vi "Update Position Simple.vi"(2 "error in (no error)":errorcluster, 3 "Time Since Last Update":dbl, 4 "Car.lvclass":refnum<class "Car.lvclass">) -> (0 "error out":errorcluster, 1 "Car.lvclass 2":refnum<class "Car.lvclass">)   [LabVIEW 2015, in "Car.lvclass"]
uses:
  Car.lvclass
  Car.lvclass/Car.ctl
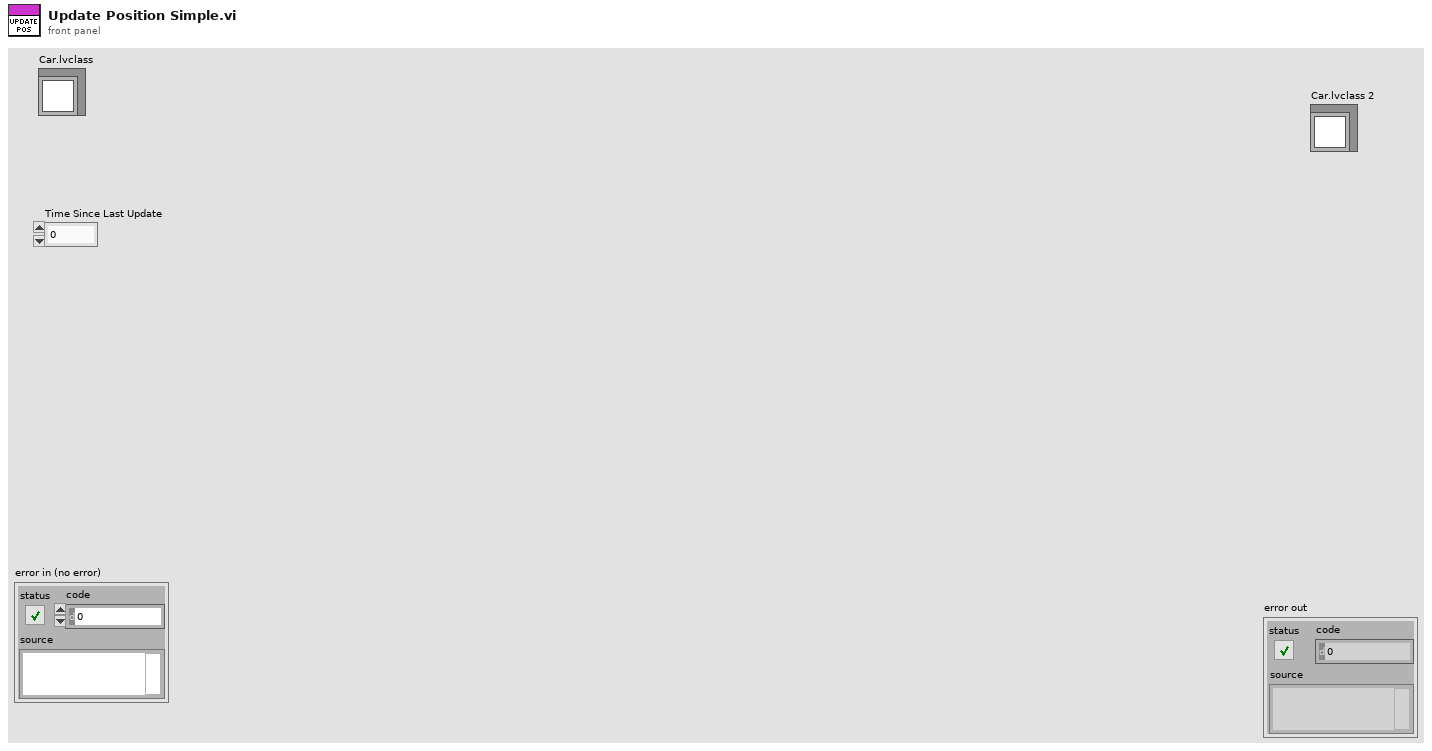
[diagram p1: front panel]
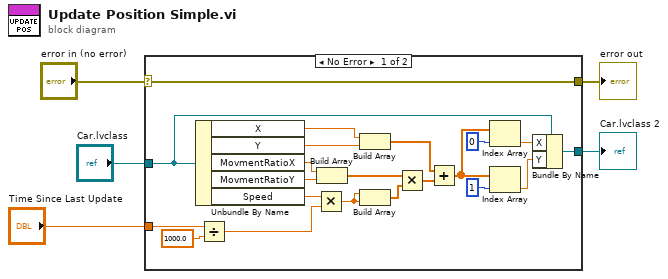
[diagram p0: block diagram]
diagram:
  n1 = case shown="No Error" "error in (no error)" {
    selector: "error in (no error)" -> [w26 w28]
    tunnel: [w26 w28] -> w4
    tunnel: [w12 w27] -> w3
    tunnel: "Car.lvclass" -> [w18 w27]
    tunnel: "Time Since Last Update" -> [w11 _]
    frame No Error {
      n2 = Unbundle By Name(w18) -> ("X"=w7:dbl, "Y"=w6:dbl, "MovmentRatioX"=w24:dbl, "MovmentRatioY"=w23:dbl, "Speed"=w8:dbl)
      n3 = Divide(x=w11, y=1000.0) -> (x/y=w9:dbl)
      n4 = Multiply(x=w8, y=w9) -> (x*y=w25:dbl)
      n5 = Build Array(w24, w23) -> (w22:dbl[])
      n6 = Build Array(w7, w6) -> (w20:dbl[])
      n7 = Build Array(w25, w25) -> (w21:dbl[])
      n8 = Multiply(x=w22, y=w21) -> (x*y=w19:dbl[])
      n9 = Add(x=w20, y=w19) -> (x+y=w13:dbl[])
      n10 = Index Array(array=w13, index=0) -> (element=w14:dbl)
      n11 = Index Array(array=w13, index=1) -> (element=w15:dbl)
      n12 = Bundle By Name(cluster=w18, "X"=w14, "Y"=w15) -> (w12:refnum<class "Car.lvclass">)
    }
    frame Error {
    }
  }
  "Car.lvclass 2" <- w3
  "error out" <- w4
